vi "Read configuration.vi"(8 "error in":errorcluster, 11 "J1939 editor node in":refnum<class "J1939 editor node.lvclass">) -> (0 "error out":errorcluster, 2 "configuration":refnum<class "NISE_CEF_serializable configuration.lvclass">, 3 "J1939 editor node out":refnum<class "J1939 editor node.lvclass">)   [LabVIEW 2013, in "J1939 editor node.lvclass"]
uses:
  J1939 editor node.lvclass
  <vilib>/NI/Configuration Framework/serializable configuration/NISE_CEF_serializable configuration.lvclass
  J1939 editor node.lvclass/J1939 editor node.ctl
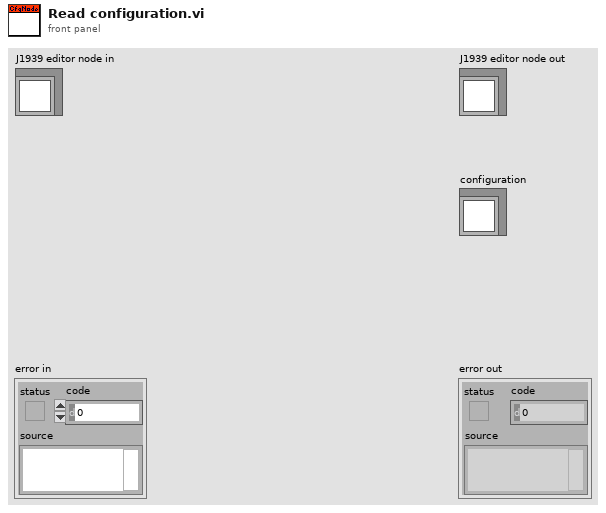
[diagram p1: front panel]
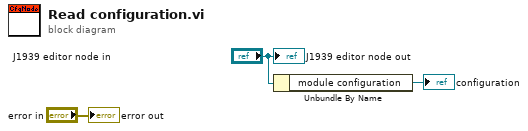
[diagram p0: block diagram]
diagram:
  n1 = Unbundle By Name("J1939 editor node in") -> ("module configuration"=→"configuration":refnum<class "J1939 configuration.lvclass">)
  "error out" <- "error in"
  "J1939 editor node out" <- "J1939 editor node in"
